vi "FGV_Stitched layout spec.vi"(8 "error in (no error)":errorcluster, 10 "Stitch layout spec":T2={"Timelapse image"={"Image position"=enum."Top left"}, "Cam 1"={"Image position"=enum."Top right"}, "Cam 2"={"Image position"=enum."Bottom left"}, "Cam 3"={"Image position"=enum."Bottom right"}, "Cam 4"={"Image position"=enum."Not used"}}, 11 "Function":T1) -> (0 "error out":errorcluster, 2 "Stitch layout spec":T2={"Timelapse image"={"Image position"=enum."Top left"}, "Cam 1"={"Image position"=enum."Top right"}, "Cam 2"={"Image position"=enum."Bottom left"}, "Cam 3"={"Image position"=enum."Bottom right"}, "Cam 4"={"Image position"=enum."Not used"}})   [LabVIEW 2013]
uses:
  Cam video sync/Typedefs/Stitch layout spec cluster.ctl
  Typedefs/Image stitching positions.ctl
  Functional Imaging Viewer/Typedefs/Get-Set-Clear Control.ctl
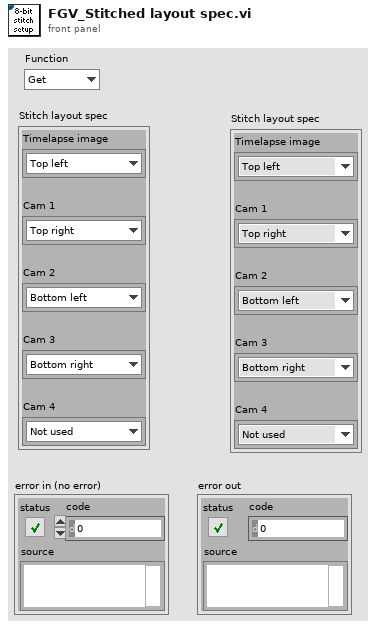
[diagram p1: front panel]
types:
  T1 = typedef "Get-Set-Clear Control.ctl" = enum16{"Get", "Set", "Clear"}
  T2 = typedef "Stitch layout spec cluster.ctl" = cluster{"Timelapse image":cluster{"Image position":T3}, "Cam 1":cluster{"Image position":T3}, "Cam 2":cluster{"Image position":T3}, "Cam 3":cluster{"Image position":T3}, "Cam 4":cluster{"Image position":T3}}
  T3 = typedef "Image stitching positions.ctl" = enum16{"Top left", "Top right", "Bottom left", "Bottom right", "Not used"}
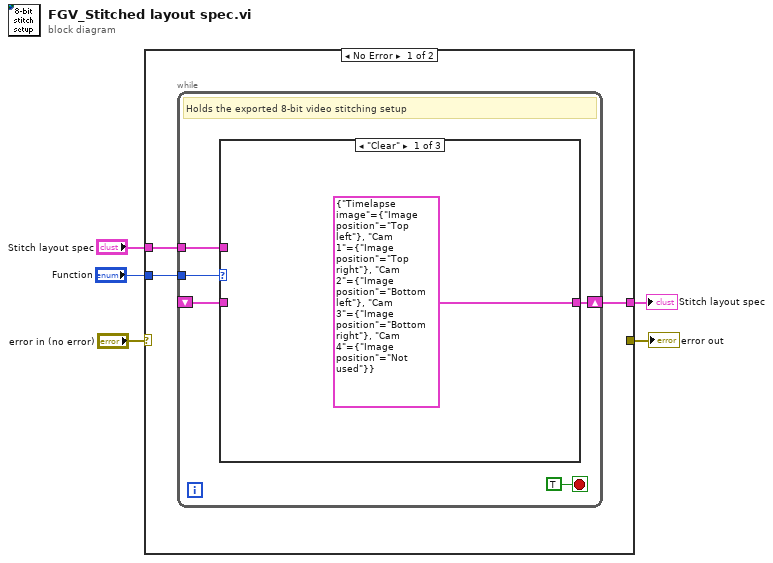
[diagram p0: block diagram]
diagram:
  n1 = case shown="No Error" "error in (no error)" {
    selector: "error in (no error)" -> [_ w17]
    tunnel: [_ w17] -> w5
    tunnel: [w8 _] -> w1
    tunnel: "Stitch layout spec" -> [w7 _]
    tunnel: "Function" -> [w6 _]
    frame No Error {
      n2 = while {
        shift-right: [w12] -> w8
        shift-left: _ -> [w11]
        tunnel: w7 -> [w10]
        tunnel: w6 -> [w9]
        stop <- TRUE stop-if-true
        # "Holds the exported 8-bit video stitching setup"
        n3 = case shown="\"Clear\"" w9 {
          tunnel: [T2 {"Timelapse image"={"Image position"=enum."Top left"}, "Cam 1"={"Image position"=enum."Top right"}, "Cam 2"={"Image position"=enum."Bottom left"}, "Cam 3"={"Image position"=enum."Bottom right"}, "Cam 4"={"Image position"=enum."Not used"}} ("Stitch layout spec") w15 w16] -> w12
          tunnel: w11 -> [_ _ w16]
          tunnel: w10 -> [_ w15 _]
          frame "Clear" {
          }
          frame "Set" {
          }
          frame "Get", Default {
          }
        }
      }
    }
    frame Error {
    }
  }
  "error out" <- w5
  "Stitch layout spec" <- w1
